vi "Calculate S and I v2.vi"(7 "current step index":i32, 11 "AC Image":dbl[][](graph)=array65x64[4160 elements]) -> ()   [LabVIEW 2014]
uses:
  <vilib>/Analysis/2dsp.llb/2D Real FFT.vi
  <vilib>/Analysis/NI_AALPro.lvlib
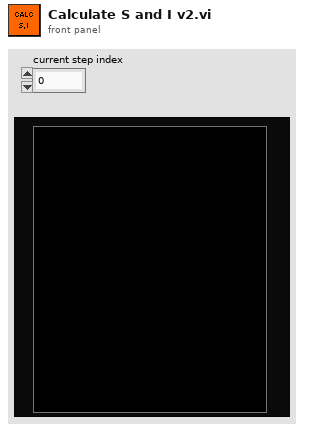
[diagram p1: front panel]
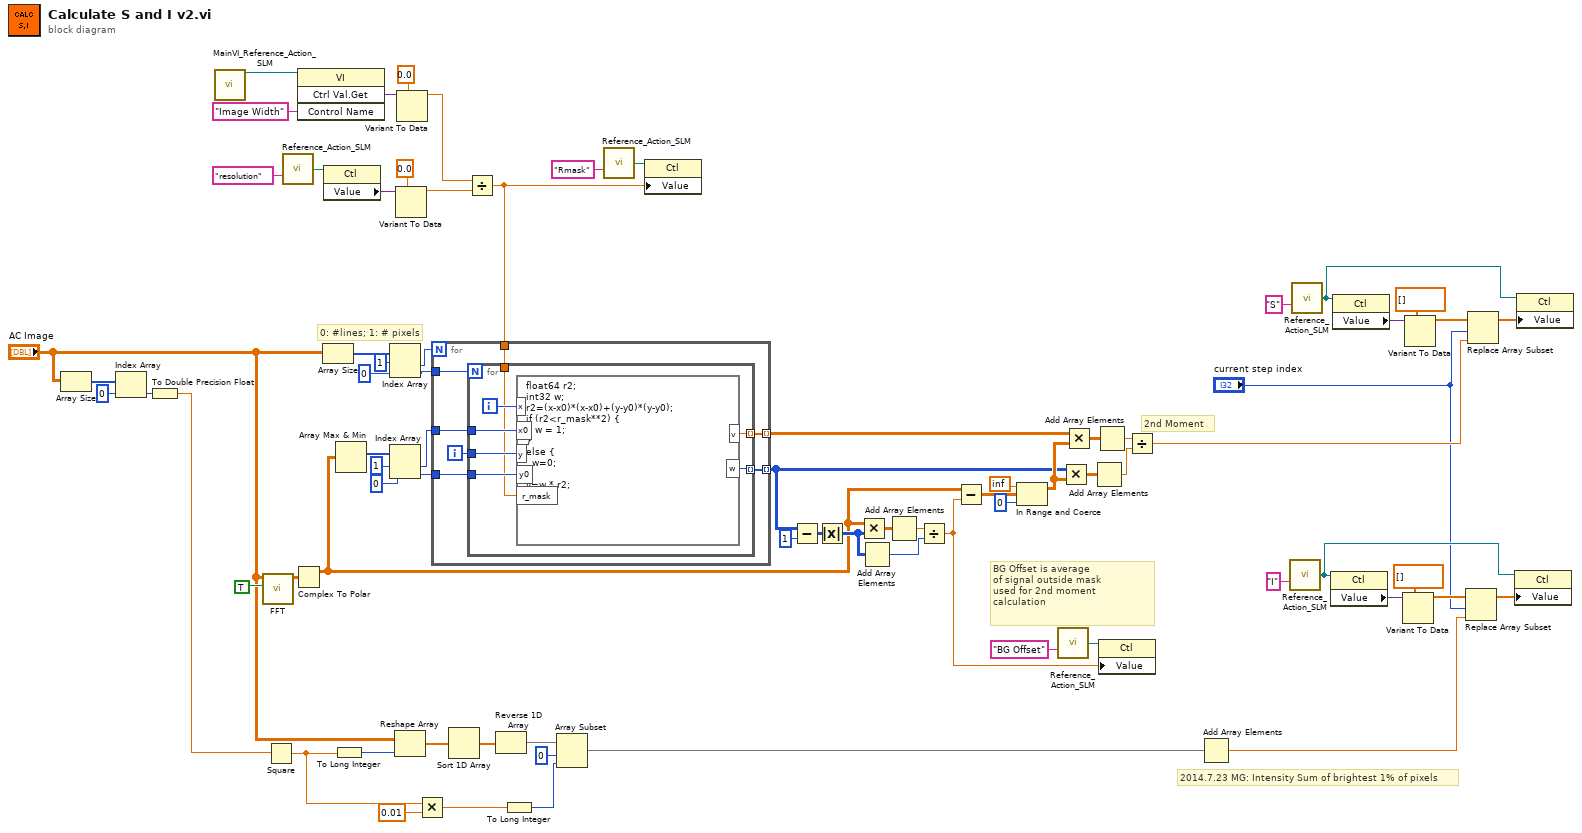
[diagram p0: block diagram]
diagram:
  # "2nd Moment"
  # "2014.7.23 MG: Intensity Sum of brightest 1% of pixels"
  # "BG Offset is average\nof signal outside mask\nused for 2nd moment\ncalculation"
  # "0: #lines; 1: # pixels"
  n1 = Array Size(array="AC Image") -> (size(s)=w46:i32[])
  n2 = Index Array(array=w46, index=0) -> (element=w44:i32)
  n3 = To Double Precision Float(number=w44) -> (double precision float=w41:dbl)
  n4 = call "MainVI_Reference_Action_SLM.vi"() -> ("VI Reference"=w29:refnum<vi>)  [unwired: 15 in]
  n5 = call-poly <vilib>:"FFT.vi"("shift?"=TRUE, "X"="AC Image") -> ("FFT {X}"=w74:cdb[][])  [unwired: 2 in, 7 out]
  n6 = Square(x=w41) -> (x^2=w38:dbl)
  n7 = call "Reference_Action_SLM.vi"("Control Name"="resolution") -> ("Ref OUT"=w25:refnum<vi>)  [unwired: 12 in, 2 out]
  n8 = Complex To Polar(r * e^(i*theta)=w74) -> (r=w47:dbl[][])  [unwired: 1 out]
  n9 = invoke class="VI" method="Ctrl Val.Get"(reference=w29, "Control Name"="Image Width") -> ("Get Control Value Variant"=w31:variant)  [unwired: 2 in, 3 out]
  n10 = Array Size(array="AC Image") -> (size(s)=w60:i32[])
  n11 = property class="Ctl"(reference=w25) -> ("Value"=w24:variant)  [unwired: 1 in, 2 out]
  n12 = To Long Integer(number=w38) -> (32bit integer=w42:i32)
  n13 = Array Max & Min(array=w47) -> (max index (indices)=w73:i32[])  [unwired: 3 out]
  n14 = Index Array(array=w60, index #1=1 ("index"), index #2=0 ("index")) -> (element #1=w57:i32, element #2=w58:i32)
  n15 = Index Array(array=w73, index #1=1 ("index"), index #2=0 ("index")) -> (element #1=w70:i32, element #2=w69:i32)
  n16 = Reshape Array("AC Image", w42) -> (w40:dbl[])
  n17 = Variant To Data(type=0.0, Variant=w24) -> (data=w22:dbl)  [unwired: 1 in, 1 out]
  n18 = Variant To Data(type=0.0, Variant=w31) -> (data=w27:dbl)  [unwired: 1 in, 1 out]
  n19 = Multiply(x=w38, y=0.01) -> (x*y=w34:dbl)
  n20 = Sort 1D Array(array=w40) -> (sorted array=w39:dbl[])
  n21 = Divide(x=w27, y=w22) -> (x/y=w19:dbl)
  n22 = for {
    N: w57 -> [_]
    tunnel: w58 -> [w82]
    tunnel: w70 -> [w81]
    tunnel: w69 -> [w80]
    tunnel: [w79] -> w68 mode=indexing
    tunnel: [w77] -> w48 mode=indexing
    tunnel: w19 -> [w76]
    i -> [w78]
    n23 = for {
      N: w82 -> [_]
      tunnel: w81 -> [w87]
      tunnel: w80 -> [w85]
      tunnel: [w89] -> w79 mode=indexing
      tunnel: w78 -> [w86]
      tunnel: [w84] -> w77 mode=indexing
      tunnel: w76 -> [w83]
      i -> [w88]
      n24 = formula code="float64 r2;\nint32 w;\nr2=(x-x0)*(x-x0)+(y-y0)*(y-y0);\nif (r2<r_mask**2) {\n   w = 1;\n}\nelse {\n  w=0;\n}\nv=w * r2;"("x"=w88, "x0"=w87, "y"=w86, "y0"=w85, "r_mask"=w83) -> ("v"=w89:dbl, "w"=w84:i32)
    }
  }
  n25 = Reverse 1D Array(array=w39) -> (reversed array=w36:dbl[])
  n26 = To Long Integer(number=w34) -> (32bit integer=w33:i32)
  n27 = Array Subset(array=w36, index=0, length=w33) -> (w32:dbl[])
  n28 = call "Reference_Action_SLM.vi"("Control Name"="Rmask") -> ("Ref OUT"=w20:refnum<vi>)  [unwired: 12 in, 2 out]
  n29 = property class="Ctl"(reference=w20, "Value"=w19) -> ()  [unwired: 1 in, 2 out]
  n30 = Subtract(x=w48, y=i8 1) -> (x-y=w54:i32[][])
  n31 = Absolute Value(x=w54) -> (abs(x)=w49:i32[][])
  n32 = Multiply(x=w47, y=w49) -> (x*y=w52:dbl[][])
  n33 = Add Array Elements(numeric array=w49) -> (sum=w50:i32)
  n34 = Add Array Elements(numeric array=w52) -> (sum=w51:dbl)
  n35 = Divide(x=w51, y=w50) -> (x/y=w16:dbl)
  n36 = Subtract(x=w47, y=w16) -> (x-y=w63:dbl[][])
  n37 = In Range and Coerce(upper limit=inf, x=w63, lower limit=0) -> (coerced(x)=w53:dbl[][])  [unwired: 1 out]
  n38 = call "Reference_Action_SLM.vi"("Control Name"="BG Offset") -> ("Ref OUT"=w17:refnum<vi>)  [unwired: 12 in, 2 out]
  n39 = Multiply(x=w48, y=w53) -> (x*y=w56:dbl[][])
  n40 = Multiply(x=w68, y=w53) -> (x*y=w67:dbl[][])
  n41 = Add Array Elements(numeric array=w56) -> (sum=w66:dbl)
  n42 = Add Array Elements(numeric array=w67) -> (sum=w65:dbl)
  n43 = property class="Ctl"(reference=w17, "Value"=w16) -> ()  [unwired: 1 in, 2 out]
  n44 = Divide(x=w65, y=w66) -> (x/y=w9:dbl)
  n45 = Add Array Elements(numeric array=w32) -> (sum=w1:dbl)
  n46 = call "Reference_Action_SLM.vi"("Control Name"="I") -> ("Ref OUT"=w5:refnum<vi>)  [unwired: 12 in, 2 out]
  n47 = call "Reference_Action_SLM.vi"("Control Name"="S") -> ("Ref OUT"=w12:refnum<vi>)  [unwired: 12 in, 2 out]
  n48 = property class="Ctl"(reference=w5) -> ("Value"=w7:variant)  [unwired: 1 in, 2 out]
  n49 = property class="Ctl"(reference=w12) -> ("Value"=w14:variant)  [unwired: 1 in, 2 out]
  n50 = Variant To Data(type=dbl[] [] ("Ab Corr VI.S"), Variant=w7) -> (data=w4:dbl[])  [unwired: 1 in, 1 out]
  n51 = Variant To Data(type=dbl[] [] ("Ab Corr VI.S"), Variant=w14) -> (data=w11:dbl[])  [unwired: 1 in, 1 out]
  n52 = Replace Array Subset(array=w4, new element=w1, index="current step index") -> (w3:dbl[])
  n53 = Replace Array Subset(array=w11, new element=w9, index="current step index") -> (w10:dbl[])
  n54 = property class="Ctl"(reference=w5, "Value"=w3) -> ()  [unwired: 1 in, 2 out]
  n55 = property class="Ctl"(reference=w12, "Value"=w10) -> ()  [unwired: 1 in, 2 out]
